vi "Lift Control.vi"(6 "bottom":bool, 7 "top":bool, 8 "Stall Speed":dbl, 10 "Motor":dbl, 11 "Enum":T1) -> (3 "bottom switch on":bool)   [LabVIEW 2014]
uses:
  TypeDefs/SRE Enum.ctl
  <vilib>/Rock Robotics/SystemInterfaces/DIO/FPGA_DIOPWMChannel.ctl
  <vilib>/Rock Robotics/WPI/MotorControl/WPI_MotorControlOpen Talon.vi
  Text Variable VIs/Read Number Variable.vi
panel:
  in  "Pot":dbl
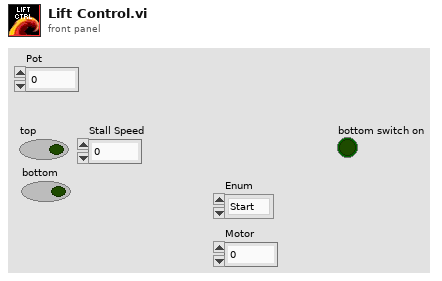
[diagram p1: front panel]
types:
  T1 = typedef "SRE Enum.ctl" = enum16{"Start", "Run", "End"}
  T2 = typedef "FPGA_DIOPWMChannel.ctl" = enum8{"PWM 0", "PWM 1", "PWM 2", "PWM 3", "PWM 4", "PWM 5", "PWM 6", "PWM 7", "PWM 8", "PWM 9", "PWM MXP 0", "PWM MXP 1", "PWM MXP 2", "PWM MXP 3", "PWM MXP 4", "PWM MXP 5", "PWM MXP 6", "PWM MXP 7", "PWM MXP 8", "PWM MXP 9", "Invalid"}
  T3 = typedef "WPI_MotorControlDeviceRef.ctl" = cluster{"DeviceStatus":errorcluster, "Type":T4, "PWM":cluster{"Controller":T5, "PWM Channel":T2, "DeadBand":T6}, "CAN":cluster{"Device Number":u8, "Control Mode":T7, "Semaphore":T8, "Max Vout":dbl, "TalonSRX Control Mode":T9}, "Invert":bool, "TransformRef":T10, "InvTransformRef":T10}
  T4 = typedef "WPI_MotorControlType.ctl" = enum16{"PWM", "CAN", "CANTalonSRX"}
  T5 = typedef "FPGA_TypedefDigitalModule.ctl" = enum16{"Controller 1"}
  T6 = typedef "WPI_PWMDeadband.ctl" = cluster{"Name":string, "maxPositivePwm":i32, "minPositivePwm":i32, "centerPwm":i32, "maxNegativePwm":i32, "minNegativePwm":i32, "angularRange":u16}
  T7 = typedef "WPI_CANJaguar_ControlMode.ctl" = enum8{"Percent VBus", "Current", "Speed", "Position", "Voltage"}
  T8 = typedef "Semaphore RefNum" = refnum<k1>
  T9 = typedef "WPI_CANTalonSRX_APIControlMode.ctl" = enum8{"Percent VBus", "Speed", "Position", "Slave", "Unchanged / Invalid"}
  T10 = typedef "WPI_PWMTransform_ConPane.ctl" = refnum<vi>
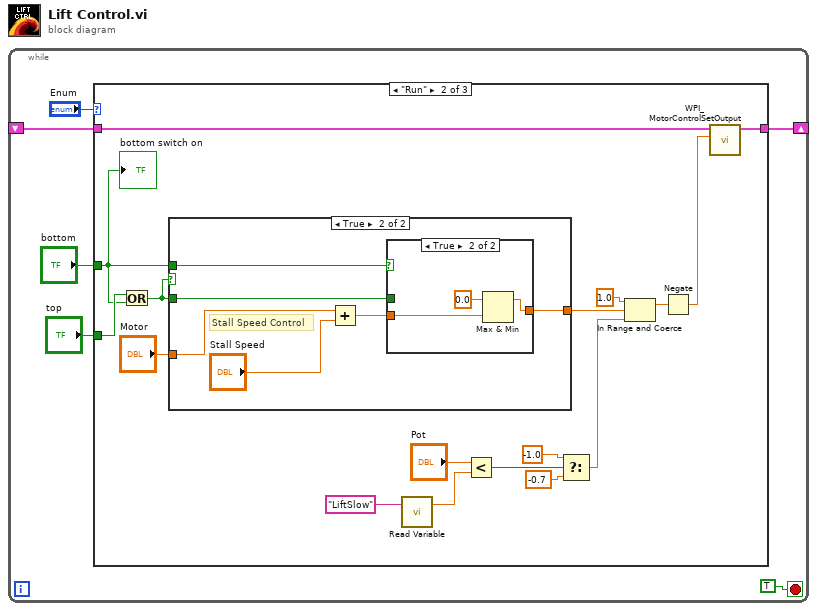
[diagram p0: block diagram]
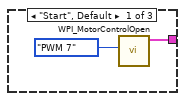
[diagram p2: hidden frame]
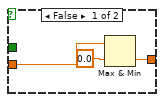
[diagram p4: hidden frame]
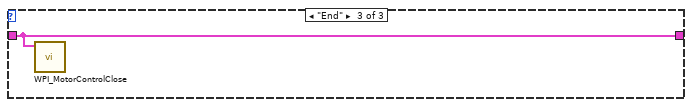
[diagram p5: hidden frame]
diagram:
  n1 = while {
    shift-right: [w5] -> _
    shift-left: _ -> [w4]
    stop <- TRUE stop-if-true
    n2 = case shown="\"Run\"" "Enum" {
      tunnel: [w8 w23 w39] -> w5
      tunnel: w4 -> [_ w22 w39]
      tunnel: "top" -> [_ w21 _]
      tunnel: "bottom" -> [_ w20 _]
      frame "Start", Default {
        n3 = call-poly <vilib>:"WPI_MotorControlOpen.vi"("PWM Channel"=FPGA_DIOPWMChannel."PWM 7") -> ("MotorControlDeviceRef"=w8:T3)  [unwired: 9 in, 1 out]
      }
      frame "Run" {
        n4 = Or(x=w21, y=w20) -> (x .or. y?=w25:bool)
        n5 = case shown="True" w25 {
          tunnel: w25 -> [_ w32]
          tunnel: "Motor" -> [w26 w29]
          tunnel: [w26 w30] -> w18
          tunnel: w20 -> [_ w31]
          frame False {
          }
          frame True {
            # "Stall Speed Control"
            n6 = Add(x=w29, y="Stall Speed") -> (x+y=w28:dbl)
            n7 = case shown="True" w31 {
              tunnel: w32 -> [_ _]
              tunnel: w28 -> [w35 w38]
              tunnel: [w33 w36] -> w30
              frame False {
                n8 = Max & Min(x=w35, y=0.0) -> (min(x,y)=w33:dbl)  [unwired: 1 out]
              }
              frame True {
                n9 = Max & Min(x=0.0, y=w38) -> (max(x,y)=w36:dbl)  [unwired: 1 out]
              }
            }
          }
        }
        n10 = call-poly "Read Variable.vi"("Name"="LiftSlow") -> ("number"=w9:dbl)  [unwired: 1 in, 1 out]
        n11 = Less?(x="Pot", y=w9) -> (x < y?=w12:bool)
        n12 = Select(t=-1.0, s=w12, f=-0.7) -> (s? t:f=w15:dbl)
        n13 = In Range and Coerce(upper limit=1.0, x=w18, lower limit=w15) -> (coerced(x)=w16:dbl)  [unwired: 1 out]
        n14 = Negate(x=w16) -> (-x=w19:dbl)
        n15 = call <vilib>:"WPI_MotorControlSetOutput.vi"("Output"=w19, "MotorControlDevRef"=w22) -> ("MotorControlDevRef"=w23:T3)  [unwired: 7 in, 2 out]
        "bottom switch on" <- w20
      }
      frame "End" {
        n16 = call <vilib>:"WPI_MotorControlClose.vi"("MotorControlDevRef"=w39) -> ()  [unwired: 10 in, 1 out]
      }
    }
  }
